vi "Tones and Noise.vi"(4 "seed":i32=-1, 6 "Fs":dbl=1000.0 format="%.2p", 7 "reset signal":bool, 8 "offset":dbl format="%.2p", 9 "noise (rms)":dbl format="%.2f", 10 "tones":T1(array[cluster])=[{"frequency"=10.0, "amplitude"=1.0, "phase"=0.0}, {"frequency"=20.0, "amplitude"=0.1, "phase"=0.0}] {"phase" format="%0.2f"; "amplitude" format="%0.2p"; "frequency" format="%0.2p"}, 11 "samples":i32=1000) -> (0 "error":i32, 3 "tones and noise":dbl[](array[numeric]) format="%.3f")   [LabVIEW 2017, in "NI_AALBase.lvlib"]
doc: "Generates an array composed of a sum of sine tones, noise, and DC offset."
uses:
  <vilib>/Analysis/NI_AALBase.lvlib
panel:
  # "Tones and Noise"
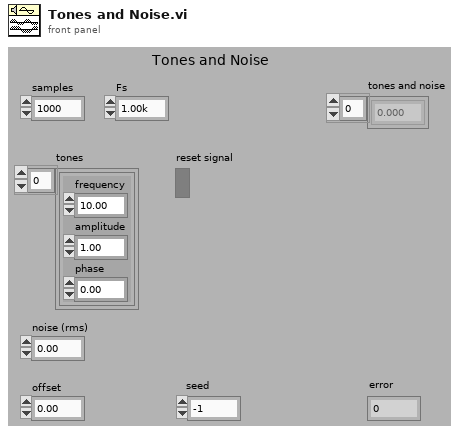
[diagram p1: front panel]
types:
  T1 = cluster{"frequency":dbl, "amplitude":dbl, "phase":dbl}[]
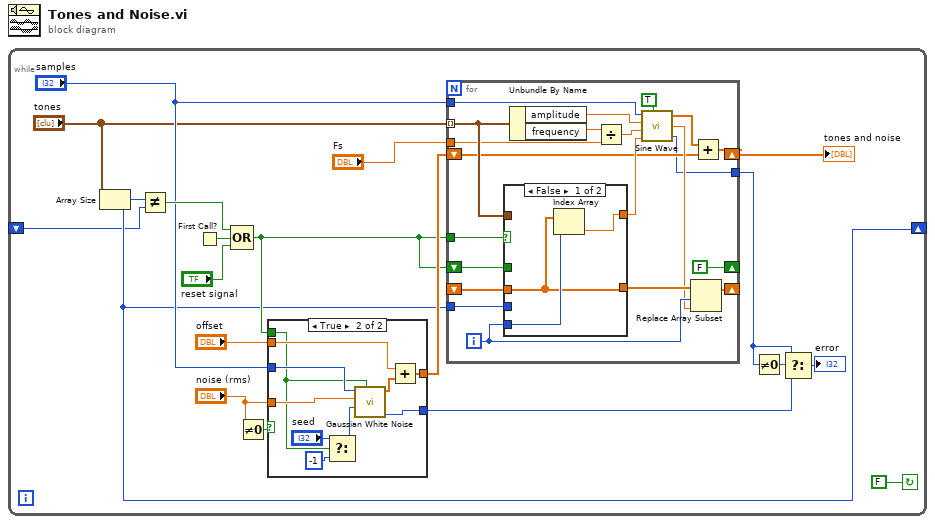
[diagram p0: block diagram]
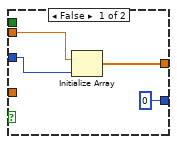
[diagram p2: hidden frame]
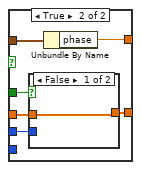
[diagram p3: hidden frame]
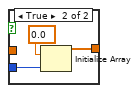
[diagram p4: hidden frame]
diagram:
  n1 = while {
    shift-right: [w4] -> _
    shift-left: _ -> [w3]
    stop <- FALSE continue-if-true
    n2 = Array Size(array="tones") -> (size(s)=w4:i32)
    n3 = Not Equal?(x=w4, y=w3) -> (x != y?=w12:bool)
    n4 = First Call?() -> (First Call?: T/F=w14:bool)
    n5 = Compound Arithmetic op=OR(w12, w14, "reset signal") -> (w13:bool)
    n6 = Not Equal To 0?(x="noise (rms)") -> (x != 0?=w17:bool)
    n7 = case shown="True" w17 {
      tunnel: "noise (rms)" -> [_ w33]
      tunnel: "offset" -> [w21 w31]
      tunnel: "samples" -> [w23 w32]
      tunnel: [w22 w30] -> w15
      tunnel: [0 ("error") w28] -> w9
      tunnel: w13 -> [_ w24]
      frame False {
        n8 = Initialize Array(w21, w23) -> (w22:dbl[])
      }
      frame True {
        n9 = Select(t="seed", s=w24, f=-1) -> (s? t:f=w25:i32)
        n10 = call <vilib>:"Gaussian White Noise.vi"("initialize?"=w24, "seed"=w25, "standard deviation"=w33, "samples"=w32) -> ("error"=w28:i32, "Gaussian noise pattern"=w29:dbl[])  [unwired: 6 in]
        n11 = Add(x=w31, y=w29) -> (x+y=w30:dbl[])
      }
    }
    n12 = for {
      tunnel: "tones" -> [w53] mode=indexing
      shift-right: [w54] -> w2
      shift-left: w15 -> [w39]
      shift-right: [w49] -> _
      shift-left: _ -> [w51]
      tunnel: "samples" -> [w37]
      tunnel: w4 -> [w43]
      tunnel: [w38] -> w10
      tunnel: w13 -> [w40]
      shift-right: [FALSE] -> _
      shift-left: w13 -> [w36]
      tunnel: "Fs" -> [w34]
      i -> [w50]
      n13 = case shown="False" w40 {
        tunnel: w53 -> [_ w63]
        tunnel: [w56 w62] -> w48
        tunnel: w43 -> [_ w60]
        tunnel: [w55 w61] -> w52
        tunnel: w51 -> [w55 w58]
        tunnel: w50 -> [w57 _]
        tunnel: w36 -> [_ w59]
        frame False {
          n14 = Index Array(array=w55, index=w57) -> (element=w56:dbl)
        }
        frame True {
          n15 = case shown="False" w59 {
            tunnel: [w64 w66] -> w61
            tunnel: w60 -> [_ w65]
            tunnel: w58 -> [w64 _]
            frame False {
            }
            frame True {
              n16 = Initialize Array(0.0 ("element"), w65) -> (w66:dbl[])
            }
          }
          n17 = Unbundle By Name(w63) -> ("phase"=w62:dbl)
        }
      }
      n18 = Unbundle By Name(w53) -> ("amplitude"=w44:dbl, "frequency"=w46:dbl)
      n19 = Divide(x=w46, y=w34) -> (x/y=w45:dbl)
      n20 = call <vilib>:"Sine Wave.vi"("samples"=w37, "amplitude"=w44, "frequency"=w45, "phase in"=w48, "reset phase"=TRUE ("reset signal")) -> ("sine wave"=w42:dbl[], "phase out"=w47:dbl, "error"=w38:i32)
      n21 = Replace Array Subset(array=w52, new element=w47, index=w50) -> (w49:dbl[])
      n22 = Add(x=w42, y=w39) -> (x+y=w54:dbl[])
    }
    "tones and noise" <- w2
    n23 = Not Equal To 0?(x=w10) -> (x != 0?=w11:bool)
    n24 = Select(t=w10, s=w11, f=w9) -> (s? t:f=→"error":i32)
  }
